vi "HEWH Trigger Draw At Time Seconds.vi"(4 "Purge Time (sec)":dbl, 6 "Full Cutout?":bool, 8 "Error In":errorcluster, 9 "Station Data Input":T1={"Sequence #"=0.0, "Cycles"=0, "Mode Setting"="", "Flow Rate (GPM)"=0.0, "Temperature (F)"=0.0, "Reset Timer"=FALSE, "Use Temp Decline Method"=FALSE, "Terminate Condition"=enum."C1-Terminate Draw @ Gallon Mark", "Condition Value #1"=0.0, "UE"=FALSE, "LE"=FALSE, "Comp"=FALSE, "Fan"=FALSE, "Test End Time (Sec)"=0.0, "Purge Until Cutout"=FALSE, "Start Conditions"=enum."Heat Source Cutout", "Condition Value #2"=0.0, "Remove Power"=FALSE, "Time"=0.0, "Check Special Cond."=enum."SC2-Check Heat Source (On-C2/Off-C1)", "Condition#"=enum."C1", "Draw Flags"=enum."N/A", "Data Processing Delay (FHD 15sec, UEF 5 Sec)"=0.0, "Test Complete"=FALSE} {"Time" format="%<%H:%M:%S>t"}, 10 "A Timer":dbl, 11 "Test Complete":bool) -> (0 "Error Out":errorcluster, 3 "Trigger Draw":bool)   [LabVIEW 2016]
uses:
  Type Definitions/PRAT Test.ctl
  Utility/Save File/File Setup (Public)/Type Definition/Save File HEWH Heating Control Mode.ctl
  Draw Water Specific/Type Definitions/Terminate Draw Conditions.ctl
  Type Definitions/HEWH Start Conditions.ctl
  Draw Water Specific/Type Definitions/Check Special Condtions.ctl
  Draw Water Specific/Type Definitions/HEWH Special Condition Check.ctl
  Type Definitions/HEWH Draw Flag ENUM.ctl
  Utility/Custom Pallet Controls/Custom Pallet String.ctl
  Utility/Type Definitions/UTILITY Notifier.ctl
  Utility/Save File/File Setup.lvlib
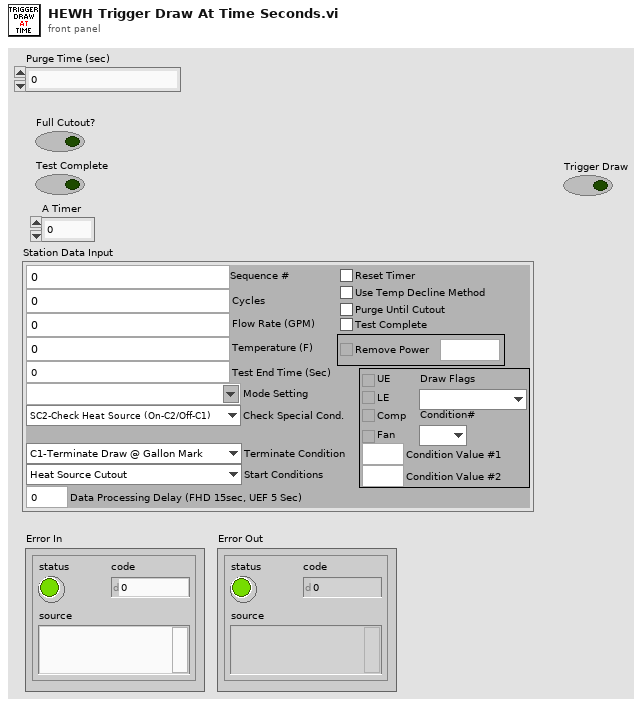
[diagram p1: front panel]
types:
  T1 = typedef "PRAT Test.ctl" = cluster{"Sequence #":dbl, "Cycles":i32, "Mode Setting":T2, "Flow Rate (GPM)":dbl, "Temperature (F)":dbl, "Reset Timer":bool, "Use Temp Decline Method":bool, "Terminate Condition":T3, "Condition Value #1":dbl, "UE":bool, "LE":bool, "Comp":bool, "Fan":bool, "Test End Time (Sec)":dbl, "Purge Until Cutout":bool, "Start Conditions":T4, "Condition Value #2":dbl, "Remove Power":bool, "Time":dbl, "Check Special Cond.":T5, "Condition#":T6, "Draw Flags":T7, "Data Processing Delay (FHD 15sec, UEF 5 Sec)":dbl, "Test Complete":bool}
  T2 = typedef "File Setup.lvlib/Save File HEWH Heating Control Mode.ctl" = string
  T3 = typedef "Terminate Draw Conditions.ctl" = enum16{"C1-Terminate Draw @ Gallon Mark", "C2-Special Last Draw (HU Test)", "C3-RTD Out <=", "C4-Mean Tank Temp <=", "C5-Decrease RTD Out (Deg F)", "C6-Time (Seconds)", "C7-Until Any Heat Source", "C8-Specific Heat Source", "C9-Do Nothing"}
  T4 = typedef "HEWH Start Conditions.ctl" = enum16{"Heat Source Cutout", "At Time (Seconds)", "Every X (Seconds)", "T2 >= X° Below Setpoint", "Seconds From Complete", "Wait for LE & Comp Cutout", "Wait for Comp Cutout", "Wait for LE Cutout", "Wait for UE Cutout"}
  T5 = typedef "Check Special Condtions.ctl" = enum16{"SC1-Do Nothing", "SC2-Check Heat Source (On-C2/Off-C1)", "SC3-Check Skip Condition", "SC4-Check Heat Source ON/Fail"}
  T6 = typedef "HEWH Special Condition Check.ctl" = enum16{"N/A", "C1", "C2", "Reset/Fail", "Skip Draw Sequence"}
  T7 = typedef "HEWH Draw Flag ENUM.ctl" = enum16{"N/A", "None(0)", "Sml(1)", "Med(2)", "SmlMed(3)", "Lrg(4)", "SmlLrg(5)", "MedLrg(6)", "SmlMedLrg(7)"}
  T8 = typedef "UTILITY Notifier.ctl" = enum16{"Set", "Read", "Release Ref"}
  T9 = typedef "Custom Pallet String.ctl" = string
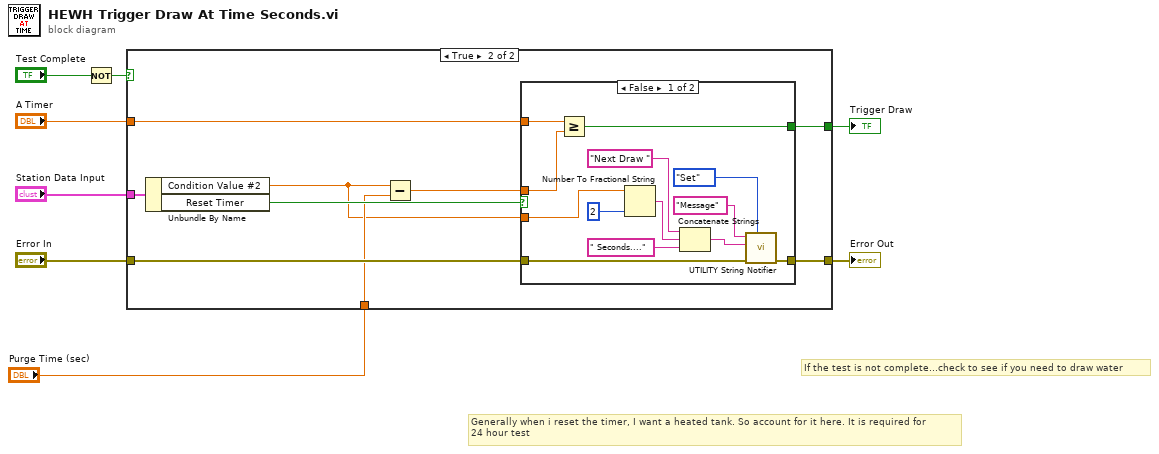
[diagram p0: block diagram]
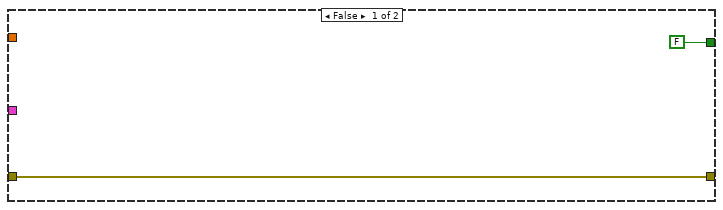
[diagram p2: hidden frame]
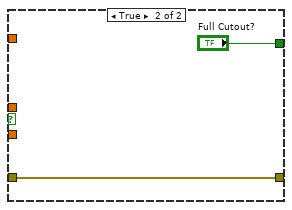
[diagram p3: hidden frame]
diagram:
  # "Generally when i reset the timer, I want a heated tank. So account for it here. It is required for \n24 hour test"
  # "If the test is not complete...check to see if you need to draw water"
  n1 = Not(x="Test Complete") -> (.not. x?=w4:bool)
  n2 = case shown="True" w4 {
    tunnel: "A Timer" -> [_ w19]
    tunnel: [FALSE w18] -> w8
    tunnel: "Station Data Input" -> [_ w17]
    tunnel: "Error In" -> [w9 w15]
    tunnel: [w9 w14] -> w2
    tunnel: "Purge Time (sec)" -> [_ w13]
    frame False {
    }
    frame True {
      n3 = Unbundle By Name(w17) -> ("Condition Value #2"=w11:dbl, "Reset Timer"=w16:bool)
      n4 = Subtract(x=w11, y=w13) -> (x-y=w12:dbl)
      n5 = case shown="False" w16 {
        tunnel: w19 -> [w32 _]
        tunnel: [w31 "Full Cutout?"] -> w18
        tunnel: w12 -> [w27 _]
        tunnel: w15 -> [w29 w33]
        tunnel: [w28 w33] -> w14
        tunnel: w11 -> [w20 _]
        frame False {
          n6 = Greater Or Equal?(x=w32, y=w27) -> (x >= y?=w31:bool)
          n7 = Number To Fractional String(number=w20, precision (6)=i16 2) -> (F-format string=w24:string)  [unwired: 2 in]
          n8 = Concatenate Strings(T9 "Next Draw " ("Message"), w24, " Seconds...." ("string")) -> (w21:string)
          n9 = call "UTILITY String Notifier.vi"("Status"=UTILITY_Notifier."Set", "error in (no error)"=w29, "Set Status"=w21, "name (unnamed)"="Message") -> ("error out"=w28:errorcluster)  [unwired: 6 in, 1 out]
        }
        frame True {
        }
      }
    }
  }
  "Trigger Draw" <- w8
  "Error Out" <- w2
